vi "Generate Message with Arguments.vi"(11 "XML String":string) -> (3 "Message with Arguments":string)   [LabVIEW 2015, in "NI_AWS_Core.lvlib" / "HTTP Request.lvclass"]
uses:
  HTTP Request.lvclass
  XML Parsing/NI_XML Parsing.lvlib
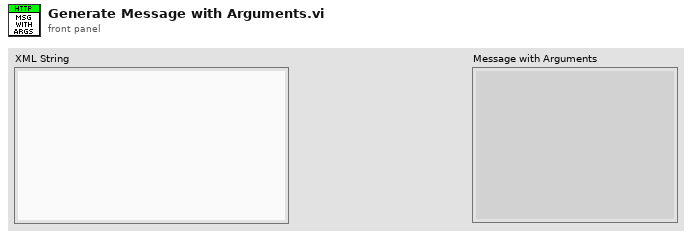
[diagram p1: front panel]
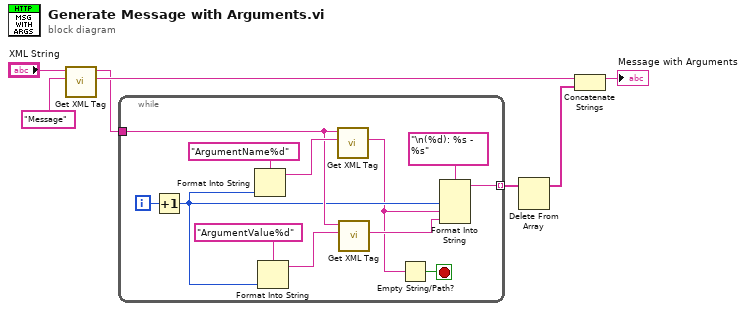
[diagram p0: block diagram]
diagram:
  n1 = call "Get XML Tag.vi"("Tag name"="Message", "XML String in"="XML String") -> ("Tag value"=w7:string, "XML String dup"=w3:string)  [unwired: 5 in, 3 out]
  n2 = while {
    tunnel: w3 -> [w14]
    tunnel: [w10] -> w2 mode=indexing
    i -> [w19]
    stop <- w8 stop-if-true
    n3 = Increment(x=w19) -> (x+1=w12:i32)
    n4 = Format Into String(format string="ArgumentName%d", w12) -> (resulting string=w17:string)  [unwired: 2 in, 1 out]
    n5 = Format Into String(format string="ArgumentValue%d", w12) -> (resulting string=w15:string)  [unwired: 2 in, 1 out]
    n6 = call "Get XML Tag.vi"("Tag name"=w17, "XML String in"=w14) -> ("Tag value"=w9:string)  [unwired: 5 in, 4 out]
    n7 = call "Get XML Tag.vi"("Tag name"=w15, "XML String in"=w14) -> ("Tag value"=w11:string)  [unwired: 5 in, 4 out]
    n8 = Empty String/Path?(string/path=w9) -> (empty?=w8:bool)
    n9 = Format Into String(format string="\n(%d): %s - %s", w12, w9, w11) -> (resulting string=w10:string)  [unwired: 2 in, 1 out]
  }
  n10 = Delete From Array(array=w2) -> (array with subset deleted=w1:string[])  [unwired: 2 in, 1 out]
  n11 = Concatenate Strings(w7, w1) -> (→"Message with Arguments":string)
